vi "Test 1 One Arrangement Two Counts.vi"(8 "error in (no error)":errorcluster, 11 "Test Case In":refnum<class "Tests.lvclass">) -> (0 "error out":errorcluster, 3 "Test Case Out":refnum<class "Tests.lvclass">)   [LabVIEW 2021, in "Tests.lvclass"]
uses:
  Tests.lvclass
  Tests.lvclass/Tests.ctl
  4993e8ee-a06a-463a-9684-69129f64d5ce.vi
  Proto/Group.lvclass
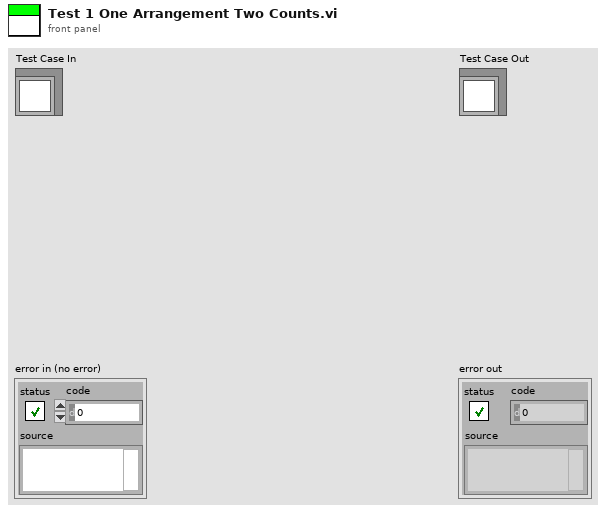
[diagram p1: front panel]
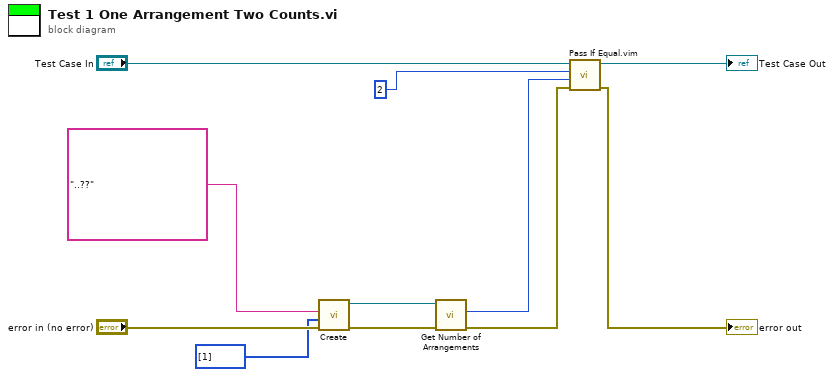
[diagram p0: block diagram]
diagram:
  n1 = call "Create.vi"("error in (no error)"="error in (no error)", "Group Sizes"=i64[] [1], "Input"="..??") -> ("error out"=w8:errorcluster, "Group Out"=w6:refnum<class "Group.lvclass">)  [unwired: 7 in]
  n2 = call "Get Number of Arrangements.vi"("error in (no error)"=w8, "Proto in"=w6) -> ("error out"=w7:errorcluster, "Arrangements"=w4:u64)  [unwired: 7 in, 1 out]
  n3 = call "Pass If Equal.vim"("error in (no error)"=w7, "Actual"=w4, "Expected"=u64 2 ("Arrangements"), "LUnit Test Case In"="Test Case In") -> ("error out"=→"error out":errorcluster, "LUnit Test Case Out"=→"Test Case Out":refnum<class "Tests.lvclass">)  [unwired: 6 in]
